vi "Log DIPS.vi"(8 "error in (no error)":errorcluster, 9 "HBDevRef":T2, 10 "Auto Mode":T1, 11 "Boolean Array":bool[](array[boolean])) -> (0 "error out":errorcluster)   [LabVIEW 2016]
uses:
  <vilib>/Rock Robotics/WPI/SerialPort/WPI_SerialPortRef.ctl
  AutoModes.ctl
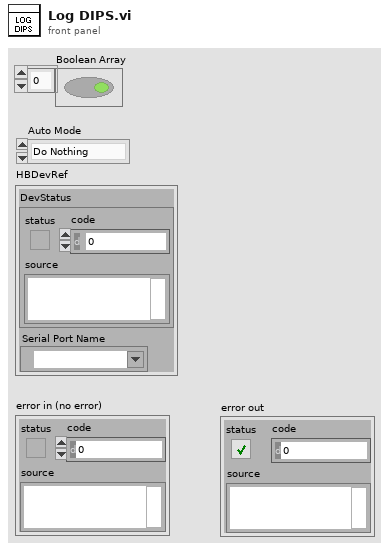
[diagram p1: front panel]
types:
  T1 = typedef "AutoModes.ctl" = enum16{"Do Nothing", "Cross Baseline", "Gear Front", "Gear Left", "Gear Right"}
  T2 = typedef "WPI_SerialPortRef.ctl" = cluster{"DevStatus":errorcluster, "Serial Port Name":refnum<visa-resource-name>}
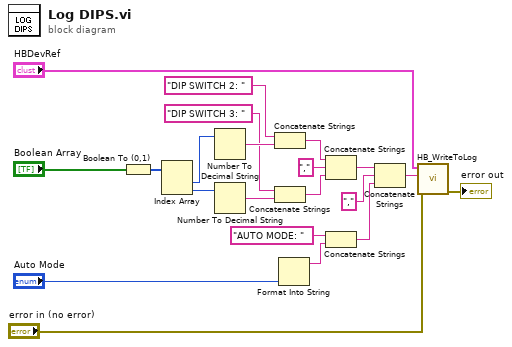
[diagram p0: block diagram]
diagram:
  n1 = Boolean To (0,1)(Boolean="Boolean Array") -> (0, 1=w3:i16[])
  n2 = Index Array(array=w3) -> (element #1=w15:i16, element #2=w14:i16)  [unwired: 2 in]
  n3 = Number To Decimal String(number=w15) -> (decimal integer string=w11:string)  [unwired: 1 in]
  n4 = Number To Decimal String(number=w14) -> (decimal integer string=w8:string)  [unwired: 1 in]
  n5 = Concatenate Strings("DIP SWITCH 2: " ("string"), w11) -> (w10:string)
  n6 = Concatenate Strings("DIP SWITCH 3: " ("string"), w8) -> (w7:string)
  n7 = Format Into String("Auto Mode") -> (resulting string=w17:string)  [unwired: 3 in, 1 out]
  n8 = Concatenate Strings(w10, "," ("string"), w7) -> (w21:string)
  n9 = Concatenate Strings("AUTO MODE: " ("string"), w17) -> (w16:string)
  n10 = Concatenate Strings(w21, "," ("string"), w16) -> (w19:string)
  n11 = call <vilib>:"HB_WriteToLog.vi"("error in (no error)"="error in (no error)", "Log string"=w19, "HBDevRef"="HBDevRef") -> ("error out"=→"error out":errorcluster)  [unwired: 7 in, 1 out]
